vi "Read Scalings.vi"(8 "error in (no error)":errorcluster, 11 "Scaling in":refnum<class "Scaling.lvclass">) -> (0 "error out":errorcluster, 2 "Scalings":T1[](array[typedef]), 3 "Scaling out":refnum<class "Scaling.lvclass">)   [LabVIEW 2018, in "Scaling.lvclass"]
doc: "Scaling.lvclass:Read Scalings.vi\n\nThis VI accesses the Scalings defined in the current configuration file.\n\nInstrument Communication Module Version 1.0\nNovember, 2017 Original Code Consulting David Thomson\n www.originalcode.com"
uses:
  Scaling.lvclass
  Scaling Def.ctl
  Scaling.lvclass/Scaling.ctl
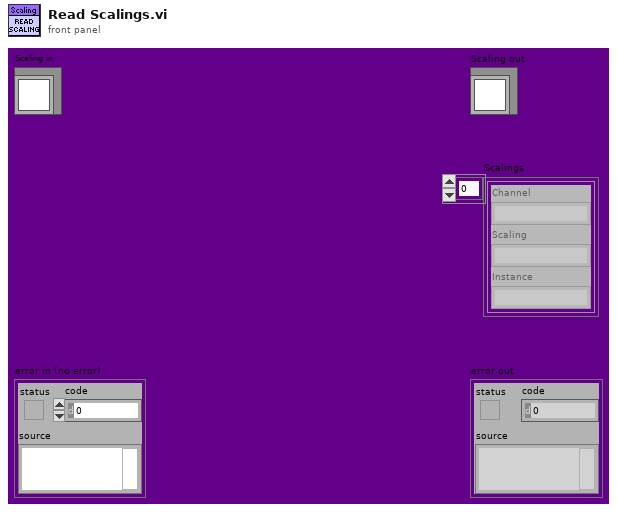
[diagram p1: front panel]
types:
  T1 = typedef "Scaling Def.ctl" = cluster{"Channel":string, "Scaling":string, "Instance":string}
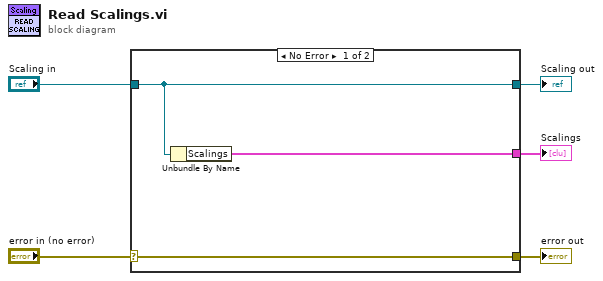
[diagram p0: block diagram]
diagram:
  n1 = case shown="No Error" "error in (no error)" {
    selector: "error in (no error)" -> [w8 w9]
    tunnel: [w8 w9] -> w4
    tunnel: [w7 w10] -> w2
    tunnel: "Scaling in" -> [w7 w10]
    tunnel: [w6 _] -> w1
    frame No Error {
      n2 = Unbundle By Name(w7) -> ("Scalings"=w6:T1[])
    }
    frame Error {
    }
  }
  "error out" <- w4
  "Scaling out" <- w2
  "Scalings" <- w1
